vi "compute_robust_adv.vi"(1 "param":T2={"Srated"=25000.0, "eta [pu]"=0.98, "model"={"in-states"={"v1"=0.0, "v2"=0.0, "SoC"=0.0}, "output"={"V"=0.0, "Zeq"=0.0, "Eeq"=0.0}}} {"model"."output"."Eeq" format="%#.6g"; "model"."output"."Zeq" format="%#.6g"; "eta [pu]" format="%#_13g"}, 2 "SoC_T":dbl, 3 "Meas":T1 {"Ud" format="%#.2f"; "P" format="%#.2f"; "Q" format="%#.2f"}) -> (0 "json-adv":string)   [LabVIEW 2021]
uses:
  General purpose/agent-variables.ctl
  General purpose/MEAS.ctl
  General purpose/robust-BA-ADV.ctl
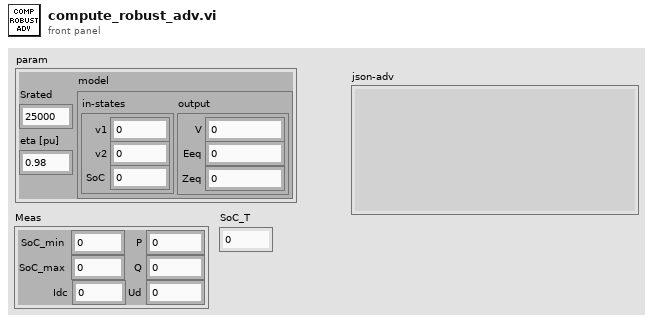
[diagram p1: front panel]
types:
  T1 = typedef "MEAS.ctl" = cluster{"P":dbl, "Q":dbl, "SoC_max":dbl, "SoC_min":dbl, "Ud":dbl, "Idc":dbl}
  T2 = typedef "agent-variables.ctl" = cluster{"Srated":dbl, "eta [pu]":dbl, "model":cluster{"in-states":cluster{"v1":dbl, "v2":dbl, "SoC":dbl}, "output":cluster{"V":dbl, "Zeq":dbl, "Eeq":dbl}}}
  T3 = typedef "robust-BA-ADV.ctl" = cluster{"Pimp":dbl, "Qimp":dbl, "Pmin":dbl, "Pmax":dbl, "Srated":dbl, "coeffP":dbl, "coeffPsquared":dbl, "SoE":dbl, "long-term":cluster{"Pmin":dbl, "Pmax":dbl}, "coeffQsquared":dbl, "coeffQ":dbl}
  T4 = typedef "cost-function.ctl" = cluster{"coeffPsquared":dbl, "coeffP":dbl, "coeffQsquared":dbl, "coeffQ":dbl}
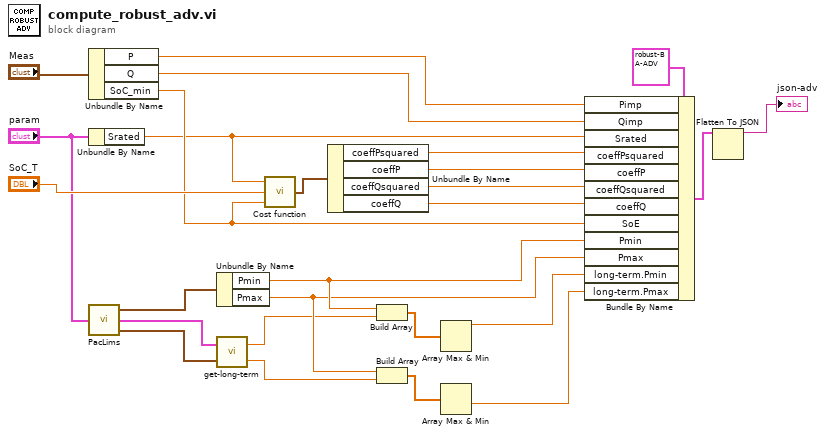
[diagram p0: block diagram]
diagram:
  n1 = Unbundle By Name("Meas") -> ("P"=w26:dbl, "Q"=w24:dbl, "SoC_min"=w19:dbl)
  n2 = Unbundle By Name("param") -> ("Srated"=w18:dbl)
  n3 = call "PacLims.vi"("param (in)"="param") -> ("PacLims"=w20:cluster{"Pmax":dbl, "Pmin":dbl}, "param (out)"=w16:T2, "Ilims"=w15:cluster{"i(Pmax)":dbl, "i(Pmin)":dbl})
  n4 = Unbundle By Name(w20) -> ("Pmin"=w11:dbl, "Pmax"=w10:dbl)
  n5 = call "get-long-term.vi"("Ilims"=w15, "param"=w16) -> ("Pmax"=w8:dbl, "Pmin"=w9:dbl)
  n6 = call "Cost function.vi"("SoC"=w19, "SoC_T"="SoC_T", "Srated"=w18) -> ("cost-function"=w5:T4)
  n7 = Unbundle By Name(w5) -> ("coeffPsquared"=w4:dbl, "coeffP"=w3:dbl, "coeffQsquared"=w2:dbl, "coeffQ"=w1:dbl)
  n8 = Build Array(w11, w9) -> (w13:dbl[])
  n9 = Build Array(w10, w8) -> (w12:dbl[])
  n10 = Array Max & Min(array=w13) -> (max value=w7:dbl)  [unwired: 3 out]
  n11 = Array Max & Min(array=w12) -> (min value=w6:dbl)  [unwired: 3 out]
  n12 = Bundle By Name(cluster=T3 {"Pimp"=0.0, "Qimp"=0.0, "Pmin"=0.0, "Pmax"=0.0, "Srated"=0.0, "coeffP"=0.0, "coeffPsquared"=0.0, "SoE"=0.0, "long-term"={"Pmin"=0.0, "Pmax"=0.0}, "coeffQsquared"=0.0, "coeffQ"=0.0} ("ADV"), "Pimp"=w26, "Qimp"=w24, "Srated"=w18, "coeffPsquared"=w4, "coeffP"=w3, "coeffQsquared"=w2, "coeffQ"=w1, "SoE"=w19, "Pmin"=w11, "Pmax"=w10, "long-term.Pmin"=w7, "long-term.Pmax"=w6) -> (w21:T3)
  n13 = Flatten To JSON(anything=w21) -> (JSON string=→"json-adv":string)  [unwired: 2 in, 1 out]
